vi "Unflatten.vi"(8 "error in":errorcluster, 10 "Buffer":u8[](array[numeric]) format="%.0x") -> (0 "error out":errorcluster, 2 "Data":T1)   [LabVIEW 2020, in "TcpReply.lvlib"]
uses:
  TcpReply.lvlib
  Data.ctl
  lv-protoc/LV-Proto/LV-Proto.lvlib
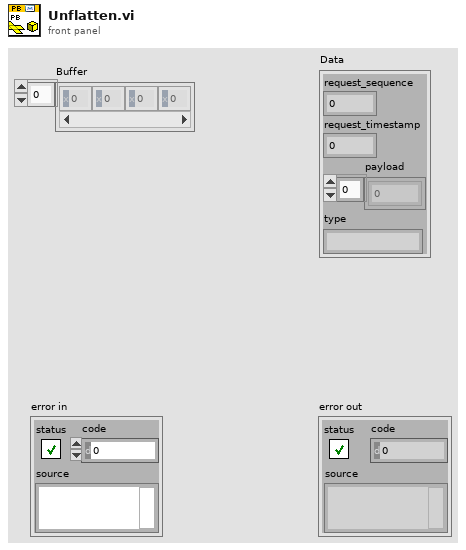
[diagram p1: front panel]
types:
  T1 = typedef "TcpReply.lvlib/Data.ctl" = cluster{"request_sequence":u32, "request_timestamp":u64, "payload":u8[], "type":string}
  T2 = typedef "LV-Proto.lvlib/Wire Type.ctl" = enum8{"VARINT", "I64", "LEN", "SGROUP (Deprecated)", "EGROUP (Deprecated)", "I32"}
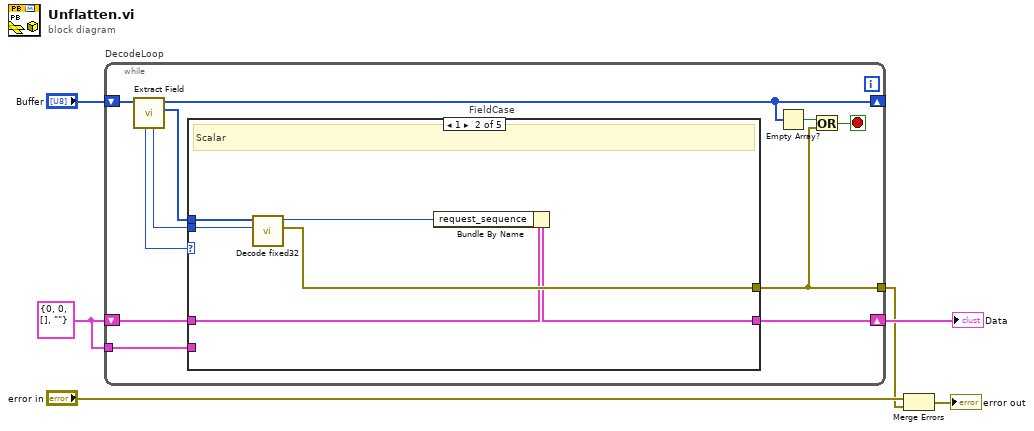
[diagram p0: block diagram]
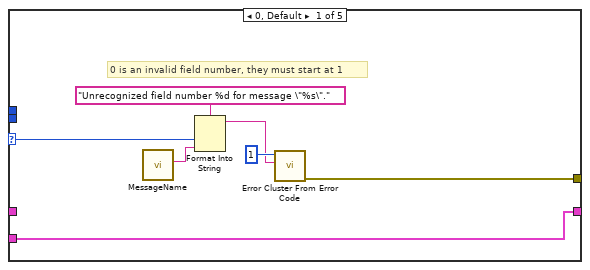
[diagram p2: hidden frame]
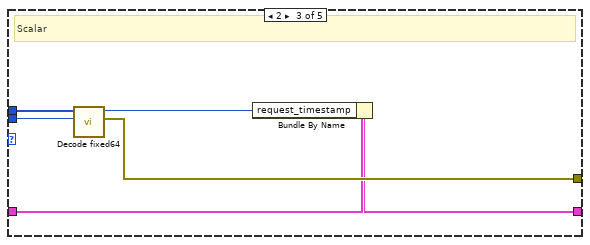
[diagram p3: hidden frame]
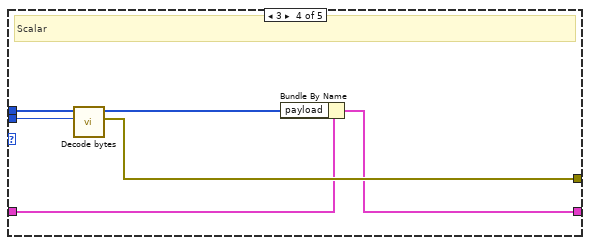
[diagram p4: hidden frame]
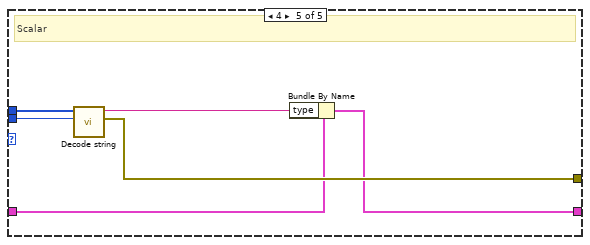
[diagram p5: hidden frame]
diagram:
  w4 = T1 {"request_sequence"=0, "request_timestamp"=0, "payload"=[], "type"=""} ("Data")
  n1 = while "DecodeLoop" {
    shift-right: [w16] -> _
    shift-left: "Buffer" -> [w17]
    shift-right: [w9] -> w5
    shift-left: w4 -> [w15]
    tunnel: [w8] -> w2
    tunnel: w4 -> [w7]
    stop <- w11 stop-if-true
    n2 = call "Extract Field.vi"("Buffer in"=w17) -> ("Field Data"=w10:u8[], "Buffer"=w16:u8[], "Wire Type"=w13:T2, "Field Number"=w14:i32)  [unwired: 7 in]
    n3 = case "FieldCase" shown="1" w14 {
      selector: w14 -> [w23 _ _ _ _]
      tunnel: w15 -> [_ w26 w32 w38 w44]
      tunnel: w13 -> [_ w28 w34 w40 w46]
      tunnel: w10 -> [_ w29 w35 w41 w47]
      tunnel: [w19 w25 w31 w37 w43] -> w9
      tunnel: [w20 w30 w36 w42 w48] -> w8
      tunnel: w7 -> [w19 _ _ _ _]
      frame 0, Default {
        # "0 is an invalid field number, they must start at 1"
        n4 = call "MessageName.vi"() -> ("MessageName"=w18:string)  [unwired: 11 in]
        n5 = Format Into String(format string="Unrecognized field number %d for message \"%s\".", w23, w18) -> (resulting string=w21:string)  [unwired: 2 in, 1 out]
        n6 = call <vilib>:"Error Cluster From Error Code.vi"("error message (\"\")"=w21, "error code (0)"=1) -> ("error out"=w20:errorcluster)  [unwired: 7 in]
      }
      frame 1 {
        # "Scalar"
        n7 = call "Decode fixed32.vi"("Wire Type"=w28, "Data"=w29) -> ("error out"=w30:errorcluster, "fixed32"=w27:u32)  [unwired: 8 in]
        n8 = Bundle By Name(cluster=w26, "request_sequence"=w27) -> (w25:T1)
      }
      frame 2 {
        # "Scalar"
        n9 = call "Decode fixed64.vi"("Wire Type"=w34, "Data"=w35) -> ("error out"=w36:errorcluster, "fixed64"=w33:u64)  [unwired: 8 in]
        n10 = Bundle By Name(cluster=w32, "request_timestamp"=w33) -> (w31:T1)
      }
      frame 3 {
        # "Scalar"
        n11 = call "Decode bytes.vi"("Wire Type"=w40, "Data"=w41) -> ("error out"=w42:errorcluster, "bytes"=w39:u8[])  [unwired: 8 in]
        n12 = Bundle By Name(cluster=w38, "payload"=w39) -> (w37:T1)
      }
      frame 4 {
        # "Scalar"
        n13 = call "Decode string.vi"("Wire Type"=w46, "Data"=w47) -> ("error out"=w48:errorcluster, "string"=w45:string)  [unwired: 8 in]
        n14 = Bundle By Name(cluster=w44, "type"=w45) -> (w43:T1)
      }
    }
    n15 = Empty Array?(array=w16) -> (empty?=w12:bool)
    n16 = Or(x=w12, y=w8) -> (x .or. y?=w11:bool)
  }
  "Data" <- w5
  n17 = Merge Errors("error in", w2) -> (→"error out":errorcluster)
